vi "BPM-Chassis04 FPGA.vi"() -> ()   [LabVIEW 2011]
uses:
  <vilib>/rvi/eio/common/nirviEmuTemplateMethod_errors.vi
  <vilib>/eio/EIONode/EIONode.xnode
  <vilib>/eio/EIOMethodNode/EIOMethodNode.xnode
  <vilib>/rvi/Analysis/measure/butterworth/XNode/niFpgaButterworthFilter.xnode
panel:
  out "Mod1/AI1":fxp<+/-,20,5> format="%.17g"
  out "Mod2/AI3":fxp<+/-,20,5> format="%.17g"
  out "Mod2/AI2":fxp<+/-,20,5> format="%.17g"
  out "Mod2/AI1":fxp<+/-,20,5> format="%.17g"
  out "Mod2/AI0":fxp<+/-,20,5> format="%.17g"
  out "Mod1/AI3":fxp<+/-,20,5> format="%.17g"
  out "Mod1/AI2":fxp<+/-,20,5> format="%.17g"
  out "Mod1/AI0":fxp<+/-,20,5> format="%.17g"
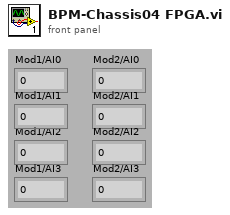
[diagram p1: front panel]
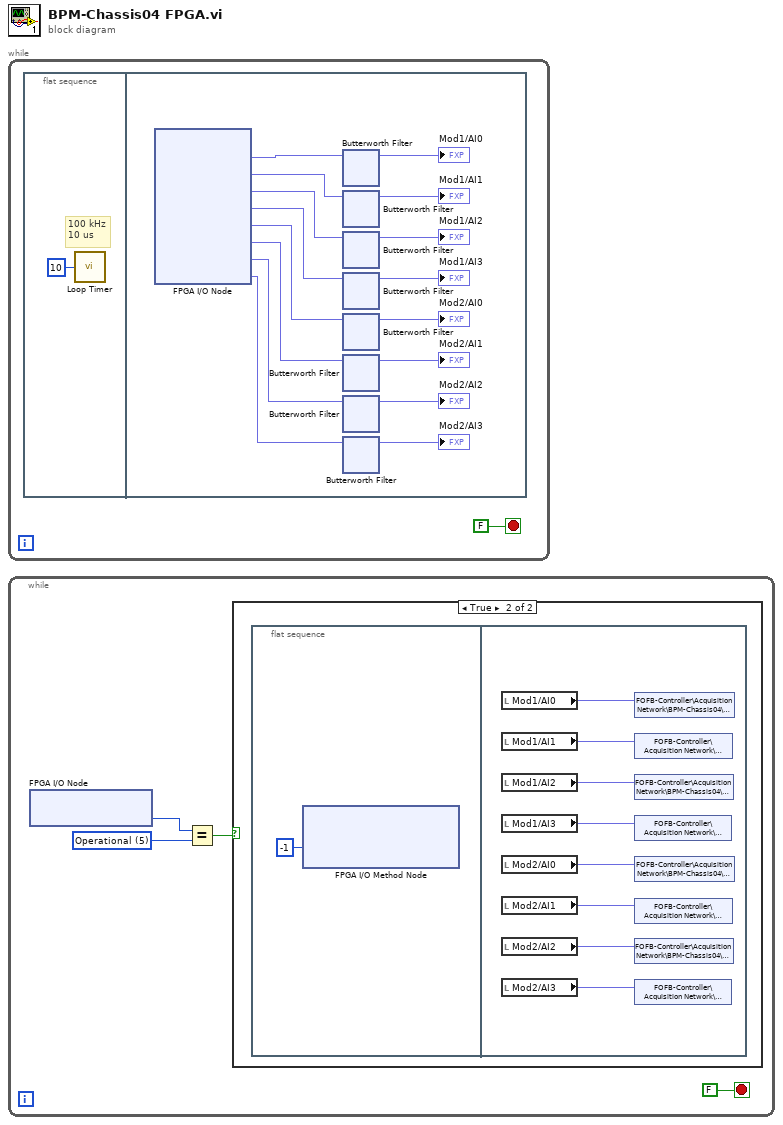
[diagram p0: block diagram]
diagram:
  n1 = while {
    stop <- FALSE stop-if-true
    n2 = flat-sequence {
      frame #0 {
        # "100 kHz\n10 us"
        n3 = call "Loop Timer"("Count(uSec)"=u8 10) -> ()  [unwired: 1 out]
      }
      frame #1 {
        n4 = xnode "FPGA I/O Node"() -> ("Mod1/AI0"=w18:fxp<+/-,20,5>, "Mod1/AI1"=w14:fxp<+/-,20,5>, "Mod1/AI2"=w13:fxp<+/-,20,5>, "Mod1/AI3"=w12:fxp<+/-,20,5>, "Mod2/AI0"=w11:fxp<+/-,20,5>, "Mod2/AI1"=w10:fxp<+/-,20,5>, "Mod2/AI2"=w9:fxp<+/-,20,5>, "Mod2/AI3"=w16:fxp<+/-,20,5>)  [unwired: 8 in, 8 out]
        n5 = xnode "Butterworth Filter"("input data"=w18) -> ("output data"=→"Mod1/AI0":fxp<+/-,20,5>)  [unwired: 2 in]
        n6 = xnode "Butterworth Filter"("input data"=w14) -> ("output data"=→"Mod1/AI1":fxp<+/-,20,5>)  [unwired: 2 in]
        n7 = xnode "Butterworth Filter"("input data"=w13) -> ("output data"=→"Mod1/AI2":fxp<+/-,20,5>)  [unwired: 2 in]
        n8 = xnode "Butterworth Filter"("input data"=w12) -> ("output data"=→"Mod1/AI3":fxp<+/-,20,5>)  [unwired: 2 in]
        n9 = xnode "Butterworth Filter"("input data"=w11) -> ("output data"=→"Mod2/AI0":fxp<+/-,20,5>)  [unwired: 2 in]
        n10 = xnode "Butterworth Filter"("input data"=w10) -> ("output data"=→"Mod2/AI1":fxp<+/-,20,5>)  [unwired: 2 in]
        n11 = xnode "Butterworth Filter"("input data"=w9) -> ("output data"=→"Mod2/AI2":fxp<+/-,20,5>)  [unwired: 2 in]
        n12 = xnode "Butterworth Filter"("input data"=w16) -> ("output data"=→"Mod2/AI3":fxp<+/-,20,5>)  [unwired: 2 in]
      }
    }
  }
  n13 = while {
    stop <- FALSE stop-if-true
    w77 = u8 5 items=["Init"=1, "PreOp"=2, "Bootstrap"=3, "SafeOp"=4, "Operational"=5]
    n14 = xnode "FPGA I/O Node"() -> ("EtherCAT State"=w76:u8)  [unwired: 1 in, 1 out]
    n15 = Equal?(x=w76, y=w77) -> (x = y?=w75:bool)
    n16 = case shown="True" w75 {
      frame False {
      }
      frame True {
        n17 = flat-sequence {
          frame #0 {
            n18 = xnode "FPGA I/O Method Node"("Timeout"=-1) -> ()  [unwired: 1 in, 2 out]
          }
          frame #1 {
            n19 = local read "Mod1/AI0"() -> (w87:fxp<+/-,20,5>)
            n20 = local read "Mod1/AI1"() -> (w85:fxp<+/-,20,5>)
            n21 = local read "Mod1/AI2"() -> (w84:fxp<+/-,20,5>)
            n22 = local read "Mod1/AI3"() -> (w83:fxp<+/-,20,5>)
            n23 = local read "Mod2/AI0"() -> (w82:fxp<+/-,20,5>)
            n24 = local read "Mod2/AI1"() -> (w81:fxp<+/-,20,5>)
            n25 = local read "Mod2/AI2"() -> (w80:fxp<+/-,20,5>)
            n26 = local read "Mod2/AI3"() -> (w86:fxp<+/-,20,5>)
            n27 = shared-variable "FOFB-Controller\\Acquisition Network\\BPM-Chassis04\\User-Defined Variables\\AMP08AH"(w87) -> ()  [unwired: 1 in, 1 out]
            n28 = shared-variable "FOFB-Controller\\Acquisition Network\\BPM-Chassis04\\User-Defined Variables\\AMP08AV"(w85) -> ()  [unwired: 1 in, 1 out]
            n29 = shared-variable "FOFB-Controller\\Acquisition Network\\BPM-Chassis04\\User-Defined Variables\\AMP08BH"(w84) -> ()  [unwired: 1 in, 1 out]
            n30 = shared-variable "FOFB-Controller\\Acquisition Network\\BPM-Chassis04\\User-Defined Variables\\AMP08BV"(w83) -> ()  [unwired: 1 in, 1 out]
            n31 = shared-variable "FOFB-Controller\\Acquisition Network\\BPM-Chassis04\\User-Defined Variables\\AMP09AH"(w82) -> ()  [unwired: 1 in, 1 out]
            n32 = shared-variable "FOFB-Controller\\Acquisition Network\\BPM-Chassis04\\User-Defined Variables\\AMP09AV"(w81) -> ()  [unwired: 1 in, 1 out]
            n33 = shared-variable "FOFB-Controller\\Acquisition Network\\BPM-Chassis04\\User-Defined Variables\\AMP09BH"(w80) -> ()  [unwired: 1 in, 1 out]
            n34 = shared-variable "FOFB-Controller\\Acquisition Network\\BPM-Chassis04\\User-Defined Variables\\AMP09BV"(w86) -> ()  [unwired: 1 in, 1 out]
          }
        }
      }
    }
  }
